vi "close.vi"(0 "object in":refnum<class "tcp_work.lvclass">, 5 "error in (no error)":errorcluster) -> (14 "object out":refnum<class "tcp_work.lvclass">, 19 "error out":errorcluster)   [LabVIEW 2016, in "tcp_work.lvclass"]
uses:
  tcp_work.lvclass
  tcp_work.lvclass/tcp_work.ctl
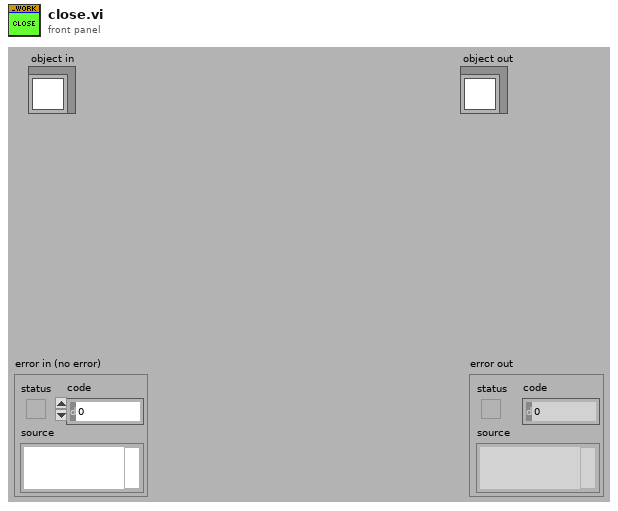
[diagram p1: front panel]
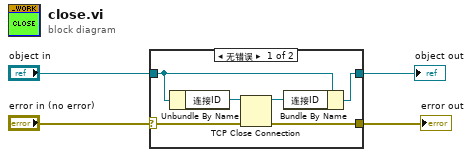
[diagram p0: block diagram]
diagram:
  n1 = case shown="无错误" "error in (no error)" {
    selector: "error in (no error)" -> [w6 w12]
    tunnel: [w5 w12] -> w3
    tunnel: [w9 w11] -> w1
    tunnel: "object in" -> [w10 w11]
    frame No Error {
      n2 = Unbundle By Name(w10) -> ("连接ID"=w8:refnum<k5>)
      n3 = TCP Close Connection(connection ID=w8, error in (no error)=w6) -> (connection ID out=w7:refnum<k5>, error out=w5:errorcluster)  [unwired: 1 in]
      n4 = Bundle By Name(cluster=w10, "连接ID"=w7) -> (w9:refnum<class "tcp_work.lvclass">)
    }
    frame Error {
    }
  }
  "error out" <- w3
  "object out" <- w1
